vi "compute_zernike_coeffs.vi"() -> ()   [LabVIEW 2020]
uses:
  ComputePhaseSet.lvclass
  HasoSlopes.lvclass
  Pupil.lvclass
  CircularPupilDetectionParams.ctl
  PupilDetectionOption.ctl
  CircularAutoDetectionOptions.ctl
  PupilDetectionMode.ctl
  ZernikeModalPrefs.ctl
  ZernikeProjectionPupilSetup.ctl
  Point2Df.ctl
  ModalCoef.lvclass
  WavefrontReconstructionMode.ctl
  WavefrontModalReconstructionType.ctl
  HasoData.lvclass
panel:
  out "Zernike pupil":i32[][](graph)
  out "Measured pupil":i32[][](graph)
  out "Zernike Coefficients":sgl[](graph)
  in  "Haso slopes file name":string="Data\\data_phase_computation.has"
  out "error out":errorcluster
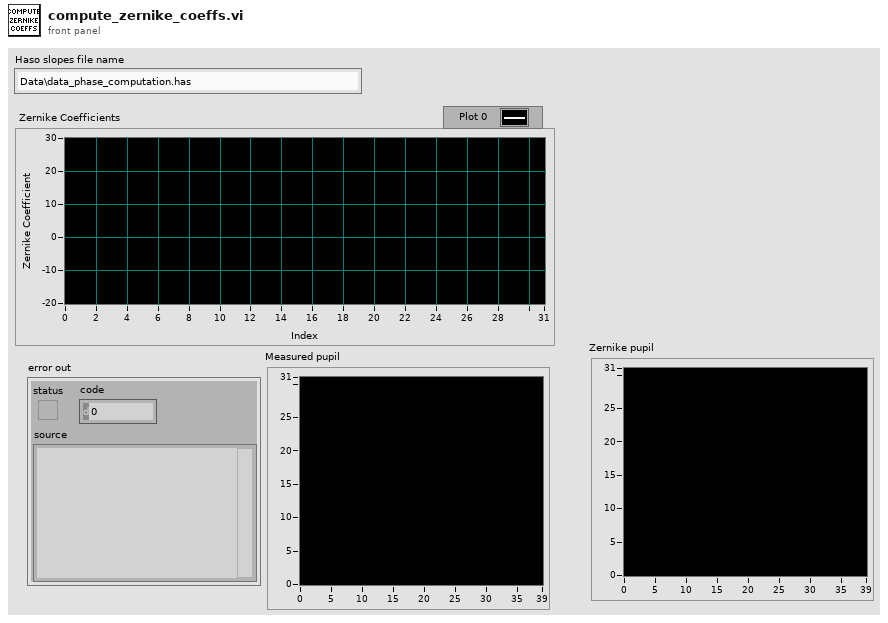
[diagram p1: front panel]
types:
  T1 = typedef "WavefrontModalReconstructionType.ctl" = enum16{"Legendre", "Zernike"}
  T2 = typedef "WavefrontReconstructionMode.ctl" = enum16{"None", "Modal_Legendre", "Modal_Zernike", "Zonal", "Modal_Zonal_Zernike", "Modal_Zonal_Legendre"}
  T3 = typedef "ZernikeModalPrefs.ctl" = cluster{"Number of coefficients":u32, "Filtered coefficients":u32[], "RMS Zernike normalization":bool, "CircularProjectionPupilDimensions":T4}
  T4 = typedef "ZernikeProjectionPupilSetup.ctl" = cluster{"Pupil center_sspp":T5, "Pupil radius_sspp":sgl}
  T5 = typedef "Point2Df.ctl" = cluster{"X":sgl, "Y":sgl}
  T6 = typedef "CircularPupilDetectionParams.ctl" = cluster{"PupilDetectionOption":T7, "AutoDetectionOption":T8, "PupilDetectionMode":T9, "CentralOccultationDetection":bool}
  T7 = typedef "PupilDetectionOption.ctl" = enum16{"Manual", "Automatic"}
  T8 = typedef "CircularAutoDetectionOptions.ctl" = enum16{"manual_radius_auto_center", "manual_center_auto_radius", "auto_radius_auto_center"}
  T9 = typedef "PupilDetectionMode.ctl" = enum16{"inscribed", "circumscribed"}
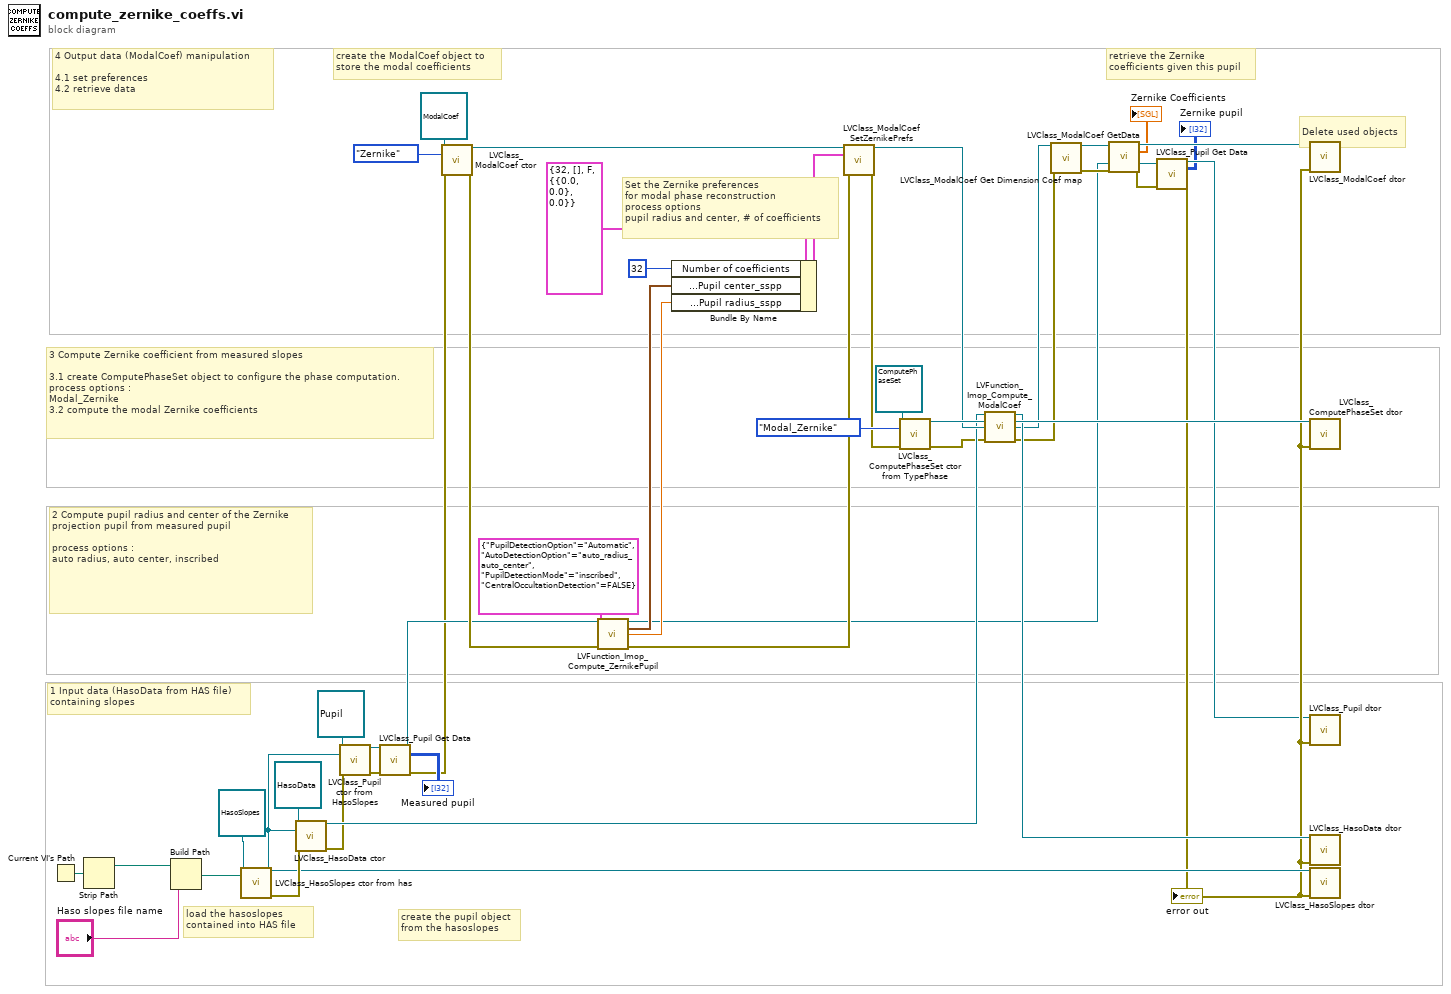
[diagram p0: block diagram]
diagram:
  # "Delete used objects"
  # "4 Output data (ModalCoef) manipulation\n\n4.1 set preferences\n4.2 retrieve data"
  # "retrieve the Zernike\ncoefficients given this pupil"
  # "create the ModalCoef object to\nstore the modal coefficients"
  # "3 Compute Zernike coefficient from measured slopes\n\n3.1 create ComputePhaseSet object to configure the phase computation.\nprocess options :\nModal_Zernike\n3.2 compute the modal Zernike coefficients"
  # "2 Compute pupil radius and center of the Zernike\nprojection pupil from measured pupil\n\nprocess options :\nauto radius, auto center, inscribed"
  # "1 Input data (HasoData from HAS file)\ncontaining slopes"
  # "Set the Zernike preferences\nfor modal phase reconstruction\nprocess options\npupil radius and center, # of coefficients"
  # "create the pupil object\nfrom the hasoslopes"
  # "load the hasoslopes\ncontained into HAS file"
  n1 = Current VI's Path() -> (path=w32:path)
  n2 = Strip Path(path=w32) -> (stripped path=w29:path)  [unwired: 1 out]
  n3 = Build Path(base path=w29, name or relative path="Haso slopes file name") -> (appended path=w30:path)
  n4 = call "LVClass_HasoSlopes ctor from has.vi"("HasoSlopes in"=refnum<class "HasoSlopes.lvclass"> refnum, ".has path"=w30) -> ("HasoSlopes out"=w16:refnum<class "HasoSlopes.lvclass">, "error out"=w19:errorcluster)  [unwired: 12 in]
  n5 = call "LVClass_HasoData ctor.vi"("HasoData in"=refnum<class "HasoData.lvclass"> refnum, "HasoSlopes.lvclass"=w16, "error in (no error)"=w19) -> ("HasoData out"=w21:refnum<class "HasoData.lvclass">, "error out"=w18:errorcluster)  [unwired: 11 in]
  n6 = call "LVClass_Pupil ctor from HasoSlopes.vi"("Pupil in"=refnum<class "Pupil.lvclass"> refnum, "HasoSlopes.lvclass"=w16, "error in (no error)"=w18) -> ("Pupil out"=w15:refnum<class "Pupil.lvclass">, "error out"=w13:errorcluster)  [unwired: 11 in]
  n7 = call "LVClass_Pupil Get Data.vi"("Pupil in"=w15, "error in (no error)"=w13) -> ("Pupil out"=w14:refnum<class "Pupil.lvclass">, "Data"=→"Measured pupil":i32[][], "error out"=w3:errorcluster)  [unwired: 11 in]
  n8 = call "LVClass_ModalCoef ctor.vi"("ModalCoef in"=refnum<class "ModalCoef.lvclass"> refnum, "TypePhase"=WavefrontModalReconstructionType."Zernike", "error in (no error)"=w3) -> ("ModalCoef out"=w23:refnum<class "ModalCoef.lvclass">, "error out"=w17:errorcluster)  [unwired: 11 in]
  n9 = call "LVFunction_Imop_Compute_ZernikePupil.vi"("Pupil.lvclass"=w14, "CircularPupilDetectionParams"=T6 {"PupilDetectionOption"=enum."Automatic", "AutoDetectionOption"=enum."auto_radius_auto_center", "PupilDetectionMode"=enum."inscribed", "CentralOccultationDetection"=FALSE}, "error in"=w17) -> ("Pupil.lvclass"=w10:refnum<class "Pupil.lvclass">, "center"=w34:T5, "radius"=w33:sgl, "error out"=w11:errorcluster)  [unwired: 9 in]
  n10 = Bundle By Name(cluster=T3 {"Number of coefficients"=32, "Filtered coefficients"=[], "RMS Zernike normalization"=FALSE, "CircularProjectionPupilDimensions"={"Pupil center_sspp"={"X"=0.0, "Y"=0.0}, "Pupil radius_sspp"=0.0}} ("ZernikeModalPrefs"), "Number of coefficients"=u32 32, "CircularProjectionPupilDimensions.Pupil center_sspp"=w34, "CircularProjectionPupilDimensions.Pupil radius_sspp"=w33) -> (w35:T3)
  n11 = call "LVClass_ModalCoef SetZernikePrefs.vi"("ModalCoef in"=w23, "ZernikeModalPrefs"=w35, "error in (no error)"=w11) -> ("ModalCoef out"=w24:refnum<class "ModalCoef.lvclass">, "error out"=w2:errorcluster)  [unwired: 11 in]
  n12 = call "LVClass_ComputePhaseSet ctor from TypePhase.vi"("ComputePhaseSet in"=refnum<class "ComputePhaseSet.lvclass"> refnum, "TypePhase"=WavefrontReconstructionMode."Modal_Zernike", "error in (no error)"=w2) -> ("ComputePhaseSet out"=w25:refnum<class "ComputePhaseSet.lvclass">, "error out"=w1:errorcluster)  [unwired: 11 in]
  n13 = call "LVFunction_Imop_Compute_ModalCoef.vi"("HasoData.lvclass"=w21, "ComputePhaseSet.lvclass"=w25, "ModalCoef.lvclass"=w24, "error constant"=w1) -> ("HasoData.lvclass (dup)"=w40:refnum<class "HasoData.lvclass">, "ComputePhaseSet.lvclass (dup)"=w41:refnum<class "ComputePhaseSet.lvclass">, "ModalCoef.lvclass (dup)"=w20:refnum<class "ModalCoef.lvclass">, "error out"=w37:errorcluster)  [unwired: 8 in]
  n14 = call "LVClass_ModalCoef Get Dimension Coef map.vi"("ModalCoef in"=w20, "error in (no error)"=w37) -> ("ModalCoef out"=w42:refnum<class "ModalCoef.lvclass">, "error out"=w38:errorcluster)  [unwired: 11 in, 1 out]
  n15 = call "LVClass_ModalCoef GetData.vi"("ModalCoef in"=w42, "Pupil.lvclass"=w10, "error in (no error)"=w38) -> ("ModalCoef out"=w39:refnum<class "ModalCoef.lvclass">, "coef"=→"Zernike Coefficients":sgl[], "Pupil.lvclass (dup)"=w8:refnum<class "Pupil.lvclass">, "error out"=w7:errorcluster)  [unwired: 8 in, 1 out]
  n16 = call "LVClass_Pupil Get Data.vi"("Pupil in"=w8, "error in (no error)"=w7) -> ("Pupil out"=w5:refnum<class "Pupil.lvclass">, "Data"=→"Zernike pupil":i32[][], "error out"=w6:errorcluster)  [unwired: 11 in]
  "error out" <- w6
  n17 = call "LVClass_ModalCoef dtor.vi"("ModalCoef in"=w39, "error in (no error)"=w6) -> ()  [unwired: 12 in, 2 out]
  n18 = call "LVClass_ComputePhaseSet dtor.vi"("ComputePhaseSet in"=w41, "error in (no error)"=w6) -> ()  [unwired: 12 in, 2 out]
  n19 = call "LVClass_Pupil dtor.vi"("Pupil in"=w5, "error in (no error)"=w6) -> ()  [unwired: 12 in, 2 out]
  n20 = call "LVClass_HasoData dtor.vi"("HasoData in"=w40, "error in (no error)"=w6) -> ()  [unwired: 12 in, 2 out]
  n21 = call "LVClass_HasoSlopes dtor.vi"("HasoSlopes in"=w16, "error in (no error)"=w6) -> ()  [unwired: 12 in, 2 out]
